vi "Example.vi"() -> ()   [LabVIEW 2018]
uses:
  Data Def/Model 3566-Setting.ctl
panel:
  out "Respond":string
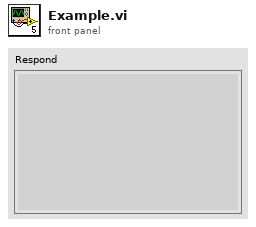
[diagram p1: front panel]
types:
  T1 = typedef "Model 3566-Setting.ctl" = cluster{"VISA Resource Name":refnum<visa-resource-name>, "ID Address":u8, "Wait For Read(ms)":u32}
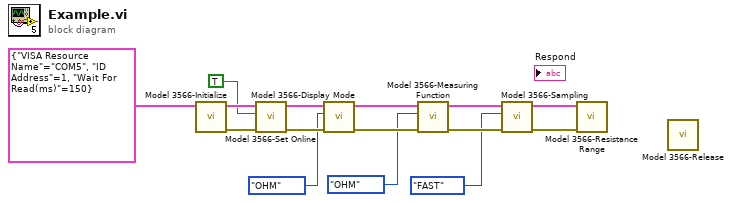
[diagram p0: block diagram]
diagram:
  n1 = call "Model 3566-Initialize.vi"("Model 3566 Setting In"=T1 {"VISA Resource Name"="COM5", "ID Address"=1, "Wait For Read(ms)"=150}) -> ("error out"=w13:errorcluster, "Model 3566 Setting Out"=w14:T1)  [unwired: 9 in]
  n2 = call "Model 3566-Set Online.vi"("error in"=w13, "Online?"=TRUE, "Model 3566 Setting In"=w14) -> ("error out"=w10:errorcluster, "Model 3566 Setting Out"=w11:T1)  [unwired: 6 in, 1 out]
  n3 = call "Model 3566-Display Mode.vi"("error in"=w10, "Function"=enum16{"OHM", "VOLT", "OHM-VOLT"}."OHM", "Model 3566 Setting In"=w11) -> ("error out"=w7:errorcluster, "Model 3566 Setting Out"=w8:T1)  [unwired: 7 in]
  n4 = call "Model 3566-Measuring Function.vi"("error in"=w7, "Mode"=enum16{"OHM", "OHM-RATIO"}."OHM", "Model 3566 Setting In"=w8) -> ("error out"=w4:errorcluster, "Model 3566 Setting Out"=w5:T1)  [unwired: 7 in]
  n5 = call "Model 3566-Sampling.vi"("error in"=w4, "Sampling"=enum16{"SLOW", "MEDIUM", "FAST"}."FAST", "Model 3566 Setting In"=w5) -> ("error out"=w1:errorcluster, "Model 3566 Setting Out"=w2:T1)  [unwired: 7 in]
  n6 = call "Model 3566-Resistance Range.vi"("error in"=w1, "Model 3566 Setting In"=w2) -> ()  [unwired: 8 in, 2 out]
  n7 = call "Model 3566-Release.vi"() -> ()  [unwired: 11 in, 1 out]
